vi "Validate Path.vi"(11 "Base Folder":path) -> (3 "Valid Path":path)   [LabVIEW 2019, in "TDMS Logger.lvlib" / "TDMS Logger.lvclass"]
uses:
  TDMS Logger.lvclass
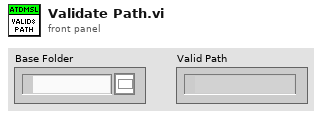
[diagram p1: front panel]
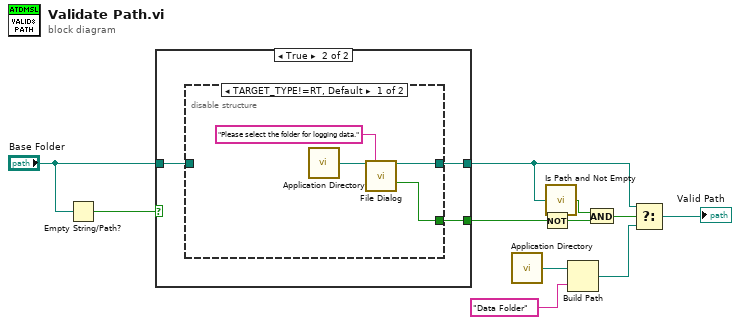
[diagram p0: block diagram]
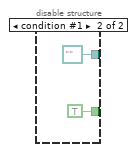
[diagram p3: hidden frame]
diagram:
  n1 = Empty String/Path?(string/path="Base Folder") -> (empty?=w7:bool)
  n2 = case shown="True" w7 {
    tunnel: [w12 w15] -> w6
    tunnel: [_ w14] -> w3
    tunnel: "Base Folder" -> [w12 w13]
    frame False {
    }
    frame True {
      n3 = disable-structure shown="TARGET_TYPE!=RT, Default" {
        disable-tunnel: [w17 path "" ("selected path")] -> w15
        disable-tunnel: [w16 TRUE ("cancelled")] -> w14
        disable-tunnel: w13 -> [_ _]
        frame condition #0 (active) {
          n4 = call <vilib>:"Application Directory.vi"() -> ("Application Directory"=w19:path)
          n5 = call "File Dialog"("start path"=w19, "prompt"="Please select the folder for logging data.") -> ("selected path"=w17:path, "cancelled"=w16:bool)  [unwired: 10 in, 2 out]
        }
        frame condition #1 {
        }
      }
    }
  }
  n6 = call <vilib>:"Application Directory.vi"() -> ("Application Directory"=w8:path)
  n7 = Not(x=w3) -> (.not. x?=w2:bool)
  n8 = call <vilib>:"Is Path and Not Empty.vi"("path"=w6) -> ("Is Path and Not Empty?"=w4:bool)  [unwired: 4 in]
  n9 = Build Path(base path=w8, name or relative path="Data Folder") -> (appended path=w10:path)
  n10 = And(x=w4, y=w2) -> (x .and. y?=w5:bool)
  n11 = Select(t=w6, s=w5, f=w10) -> (s? t:f=→"Valid Path":path)
